vi "ButtonControl.vi"(4 "SubPanel Command":T1, 5 "user event in":refnum<user-event>, 6 "MenuButtons":path[](array[path]), 7 "error in (no error)":errorcluster, 8 "SubMenuButtons":path[](array[path]), 9 "SubMenuButtonPanels":refnum<vi>[](array[refnum]), 10 "MenuButtonPanels":refnum<vi>[](array[refnum])) -> (0 "error out":errorcluster, 3 "user event Out":refnum<user-event>)   [LabVIEW 2023]
uses:
  ButtonCommands.ctl
panel:
  # "Input"
  # "Output"
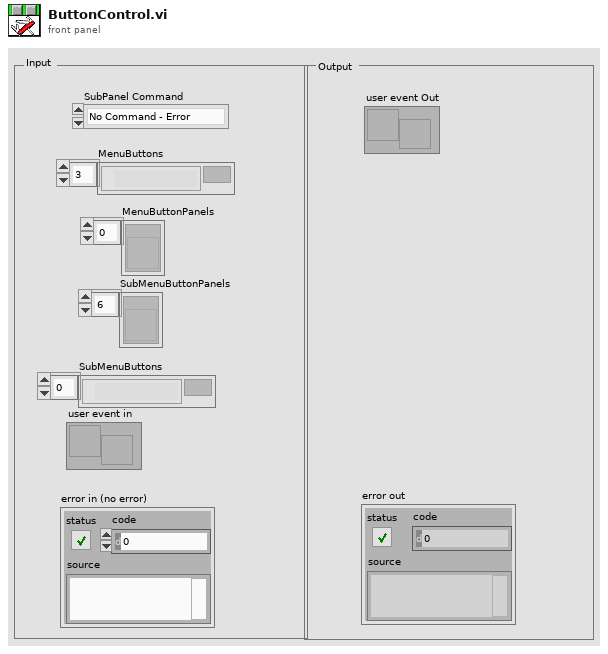
[diagram p1: front panel]
types:
  T1 = typedef "ButtonCommands.ctl" = enum16{"No Command - Error", "Load Buttons", "Remove Buttons", "Get User Events"}
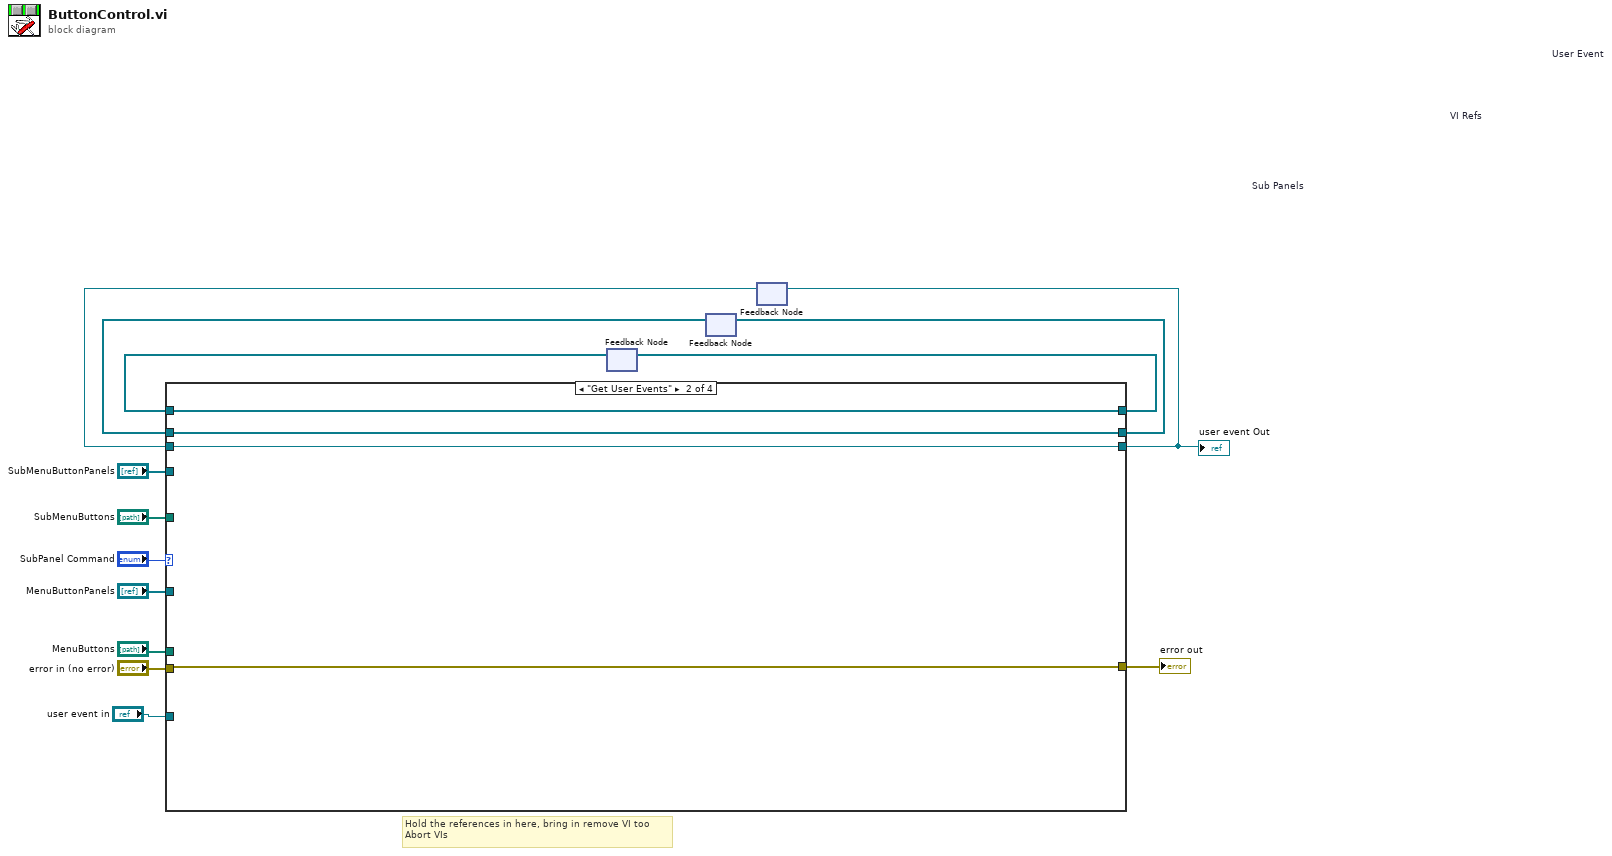
[diagram p0: block diagram]
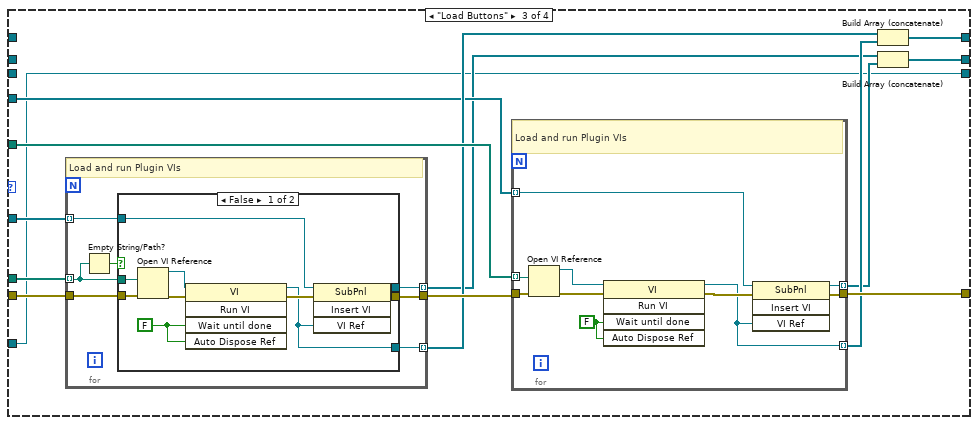
[diagram p3: hidden frame]
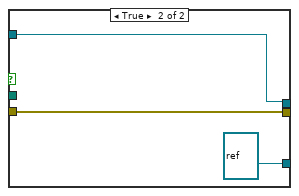
[diagram p4: hidden frame]
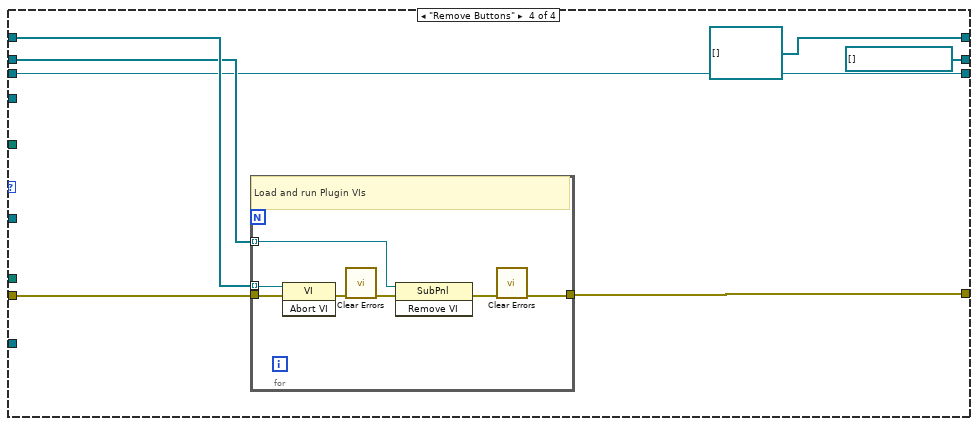
[diagram p5: hidden frame]
diagram:
  # "Hold the references in here, bring in remove VI too\nAbort VIs"
  n1 = feedback #1 "Sub Panels"() -> (w6:refnum<vi>[])  [unwired: 1 in]
  n2 = feedback #2 "VI Refs"() -> (w4:refnum<vi>[])  [unwired: 1 in]
  n3 = feedback #3 "User Event"() -> (w2:refnum<user-event>)  [unwired: 1 in]
  n4 = case shown="\"Get User Events\"" "SubPanel Command" {
    tunnel: "MenuButtons" -> [_ _ w36 _]
    tunnel: "error in (no error)" -> [w17 w21 w35 w72]
    tunnel: "MenuButtonPanels" -> [_ _ w27 _]
    tunnel: [w17 w21 w34 w73] -> w11
    tunnel: "SubMenuButtonPanels" -> [_ _ w28 _]
    tunnel: "SubMenuButtons" -> [_ _ w32 _]
    tunnel: [w18 w22 w29 refnum<vi>[] []] -> w7
    tunnel: w6 -> [w18 w22 _ w70]
    tunnel: [w16 w20 w26 refnum<vi>[] []] -> w5
    tunnel: w4 -> [w16 w20 _ w68]
    tunnel: "user event in" -> [_ _ w23 _]
    tunnel: [w15 w19 w23 w67] -> w1
    tunnel: w2 -> [w15 w19 _ w67]
    frame "No Command - Error", Default {
    }
    frame "Get User Events" {
    }
    frame "Load Buttons" {
      n5 = for {
        tunnel: w35 -> [w53]
        tunnel: [w52] -> w33
        tunnel: w36 -> [w47] mode=indexing
        tunnel: w27 -> [w51] mode=indexing
        tunnel: [w50] -> w31 mode=indexing
        tunnel: [w49] -> w24 mode=indexing
        # "Load and run Plugin VIs"
        n6 = Empty String/Path?(string/path=w47) -> (empty?=w48:bool)
        n7 = case shown="False" w48 {
          tunnel: w53 -> [w63 w65]
          tunnel: w47 -> [w62 _]
          tunnel: [w61 w65] -> w52
          tunnel: w51 -> [w60 w66]
          tunnel: [w55 refnum<vi> refnum ("type specifier VI Refnum (for type only)")] -> w50
          tunnel: [w59 w66] -> w49
          frame False {
            w54 = FALSE ("Wait Until Done")
            n8 = Open VI Reference(vi path=w62, error in (no error)=w63) -> (vi reference=w57:refnum<vi>, error out=w58:errorcluster)  [unwired: 4 in]
            n9 = invoke class="VI" method="Run VI"(reference=w57, error in=w58, "Wait until done"=w54, "Auto Dispose Ref"=w54) -> (reference out=w55:refnum<vi>, error out=w56:errorcluster)  [unwired: 1 in, 3 out]
            n10 = invoke on="Invoke Node" class="SubPnl" method="Insert VI"(reference=w60, error in=w56, "VI Ref"=w55) -> (reference out=w59:refnum<vi>, error out=w61:errorcluster)  [unwired: 1 in, 2 out]
          }
          frame True {
          }
        }
      }
      n11 = for {
        tunnel: w33 -> [w46]
        tunnel: [w44] -> w34
        tunnel: w32 -> [w45] mode=indexing
        tunnel: w28 -> [w43] mode=indexing
        tunnel: [w38] -> w30 mode=indexing
        tunnel: [w42] -> w25 mode=indexing
        w37 = FALSE ("Wait Until Done")
        # "Load and run Plugin VIs"
        n12 = Open VI Reference(vi path=w45, error in (no error)=w46) -> (vi reference=w41:refnum<vi>, error out=w40:errorcluster)  [unwired: 4 in]
        n13 = invoke class="VI" method="Run VI"(reference=w41, error in=w40, "Wait until done"=w37, "Auto Dispose Ref"=w37) -> (reference out=w38:refnum<vi>, error out=w39:errorcluster)  [unwired: 1 in, 3 out]
        n14 = invoke on="Invoke Node" class="SubPnl" method="Insert VI"(reference=w43, error in=w39, "VI Ref"=w38) -> (reference out=w42:refnum<vi>, error out=w44:errorcluster)  [unwired: 1 in, 2 out]
      }
      n15 = Build Array (concatenate)(w31, w30) -> (w29:refnum<vi>[])
      n16 = Build Array (concatenate)(w24, w25) -> (w26:refnum<vi>[])
    }
    frame "Remove Buttons" {
      n17 = for {
        tunnel: w72 -> [w77]
        tunnel: [w74] -> w73
        tunnel: w70 -> [w76] mode=indexing
        tunnel: w68 -> [w78] mode=indexing
        # "Load and run Plugin VIs"
        n18 = invoke class="VI" method="Abort VI"(reference=w76, error in=w77) -> (error out=w80:errorcluster)  [unwired: 1 in, 2 out]
        n19 = call <vilib>:"Clear Errors.vi"("error in (no error)"=w80) -> ("error out"=w75:errorcluster)  [unwired: 5 in, 1 out]
        n20 = invoke on="Invoke Node" class="SubPnl" method="Remove VI"(reference=w78, error in=w75) -> (error out=w79:errorcluster)  [unwired: 1 in, 2 out]
        n21 = call <vilib>:"Clear Errors.vi"("error in (no error)"=w79) -> ("error out"=w74:errorcluster)  [unwired: 5 in, 1 out]
      }
    }
  }
  "error out" <- w11
  "user event Out" <- w1
  n22 = feedback-in #1(w7) -> ()
  n23 = feedback-in #2(w5) -> ()
  n24 = feedback-in #3(w1) -> ()
